vi "oximentro.vi"() -> ()   [LabVIEW 2016]
uses:
  <vilib>/Utility/error.llb/whitespace.ctl
  <vilib>/Instr/_visa.llb/VISA Configure Serial Port (Instr).vi
panel:
  in  "Stop Button":bool
  in  "Listbox":i32(listbox)
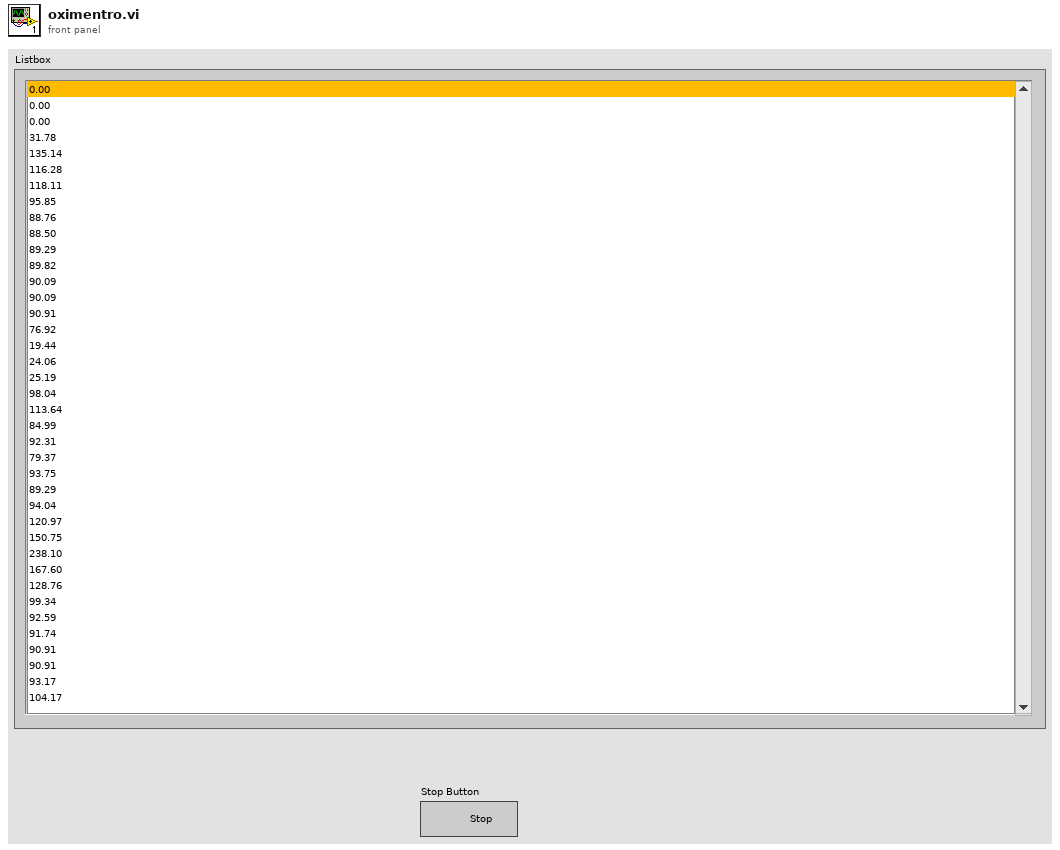
[diagram p1: front panel]
types:
  T1 = typedef "whitespace.ctl" = u16
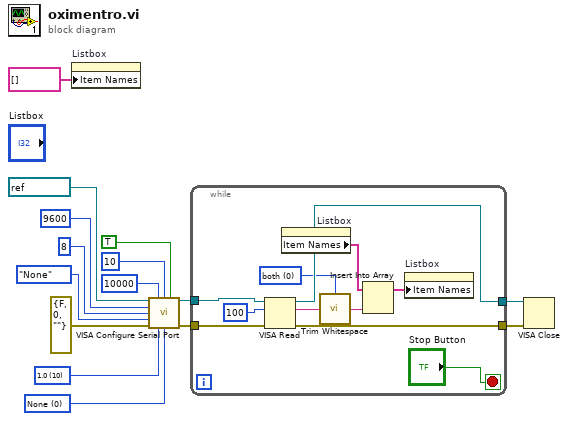
[diagram p0: block diagram]
diagram:
  w6 = u16 0 items=["None", "XON/XOFF", "RTS/CTS", "XON/XOFF & RTS/CTS", "DTR/DSR", "XON/XOFF & DTR/DSR"] ("flow control (0:none)")
  w7 = u16 10 items=["1.0"=10, "1.5"=15, "2.0"=20] ("stop bits (10: 1 bit)")
  n1 = property on="Listbox" class="LstBox (strict)"("Item Names"=string[] []) -> ()  [unwired: 2 in, 2 out]
  n2 = call-poly "VISA Configure Serial Port"("VISA resource name"=refnum<visa-resource-name> "COM6", "timeout (10sec)"=u32 10000, "termination char\n(0xA = '\\n' = LF)"=u8 10 ("termination char\n(0xA = '\\n' = LF)"), "Enable Termination\nChar (T)"=TRUE ("Enable Termination\nChar (T)"), "baud rate (9600)"=u32 9600, "data bits (8)"=u16 8, "parity (0:none)"=enum16{"None", "Odd", "Even", "Mark", "Space"}."None", "error in (no error)"=errorcluster {"status"=FALSE, "code"=0, "source"=""}, "stop bits (10: 1 bit)"=w7, "flow control (0:none)"=w6) -> ("VISA resource name out"=w5:refnum<visa-resource-name>, "error out"=w4:errorcluster)  [unwired: 4 in]
  n3 = while {
    tunnel: w5 -> [w26]
    tunnel: w4 -> [w25]
    tunnel: [w20] -> w2
    tunnel: [w19] -> w1
    stop <- "Stop Button" stop-if-true
    w16 = T1 0 items=["both", "start of string", "end of string"] ("location (both)")
    n4 = VISA Read(VISA resource name=w26, byte count=u32 100, error in (no error)=w25) -> (VISA resource name out=w20:refnum<visa-resource-name>, read buffer=w18:string, error out=w19:errorcluster)  [unwired: 1 out]
    n5 = property on="Listbox" class="LstBox (strict)"() -> ("Item Names"=w22:string[])  [unwired: 2 in, 2 out]
    n6 = call <vilib>:"Trim Whitespace.vi"("string"=w18, "location (both)"=w16) -> ("trimmed string"=w17:string)
    n7 = Insert Into Array(array=w22, new element=w17) -> (w21:string[])  [unwired: 1 in]
    n8 = property on="Listbox" class="LstBox (strict)"("Item Names"=w21) -> ()  [unwired: 2 in, 2 out]
  }
  n9 = VISA Close(VISA resource name=w2, error in (no error)=w1) -> ()  [unwired: 1 out]
